vi "Errorbar1003.vi"   [LabVIEW 2013]
uses:
  <vilib>/Heliosphere Research LLC/Advanced Plotting Toolkit/api_plotting/ErrorbarProperties.ctl
  <vilib>/Heliosphere Research LLC/Advanced Plotting Toolkit/typedefs/PlotColor.ctl
  <vilib>/Heliosphere Research LLC/Advanced Plotting Toolkit/properties/Display.ctl
  <vilib>/Heliosphere Research LLC/Advanced Plotting Toolkit/Advanced Plotting Toolkit.lvlib
types:
  T1 = typedef "Advanced Plotting Toolkit.lvlib/ErrorbarProperties.ctl" = cluster{"Color":T2, "Line Width":dbl, "Cap Size":dbl, "Display":T3}
  T2 = typedef "Advanced Plotting Toolkit.lvlib/PlotColor.ctl" = u32
  T3 = typedef "Advanced Plotting Toolkit.lvlib/Display.ctl" = cluster{"Alpha":dbl, "Z Order":dbl}
  T4 = typedef "Advanced Plotting Toolkit.lvlib/PlotID.ctl" = i32
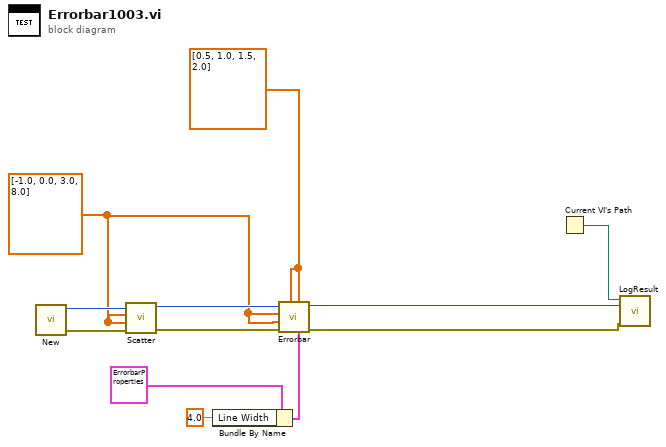
[diagram p0: block diagram]
diagram:
  w4 = dbl[] [0.5, 1.0, 1.5, 2.0] ("X Errors")
  w5 = dbl[] [-1.0, 0.0, 3.0, 8.0] ("X Data")
  n1 = call <vilib>:"New.vi"() -> ("error out"=w6:errorcluster, "Plot ID"=w9:T4)  [unwired: 10 in]
  n2 = call <vilib>:"Scatter.vi"("error in (no error)"=w6, "Y Data"=w5, "X Data"=w5, "Plot ID"=w9) -> ("error out"=w7:errorcluster, "Plot ID Out"=w8:T4)  [unwired: 6 in]
  n3 = Bundle By Name(cluster=T1 {"Color"=2147483647, "Line Width"=nan, "Cap Size"=nan, "Display"={"Alpha"=nan, "Z Order"=nan}} ("Errorbar Properties"), "Line Width"=4.0) -> (w2:T1)
  n4 = call <vilib>:"Errorbar.vi"("Properties"=w2, "Y Errors"=w4, "X Errors"=w4, "error in (no error)"=w7, "Y Data"=w5, "X Data"=w5, "Plot ID"=w8) -> ("error out"=w10:errorcluster, "Plot ID out"=w11:T4)  [unwired: 3 in]
  n5 = Current VI's Path() -> (path=w12:path)
  n6 = call "LogResult.vi"("Test Result"=w10, "Test Artifact"=w11, "VI Path"=w12) -> ()  [unwired: 9 in]
